vi "ALTS-2015 Convert Test Time format.vi"(8 "error in (no error)":errorcluster, 11 "String":string) -> (0 "error out":errorcluster, 3 "Test Time(YYYYMMDDHHMMSS)":string)   [LabVIEW 2013]
doc: "Copyright © 2005, Soliton Technologies.\nAll rights reserved."
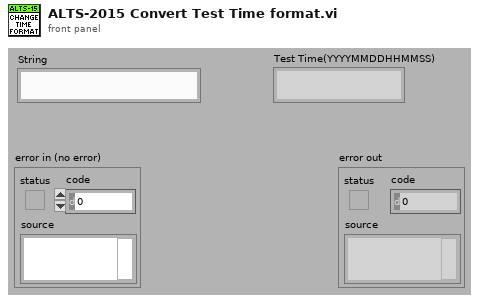
[diagram p1: front panel]
types:
  T1 = cluster{"YYYY":string, "MM":string, "DD":string, "HH":string, "Min MM":string, "SS":string}
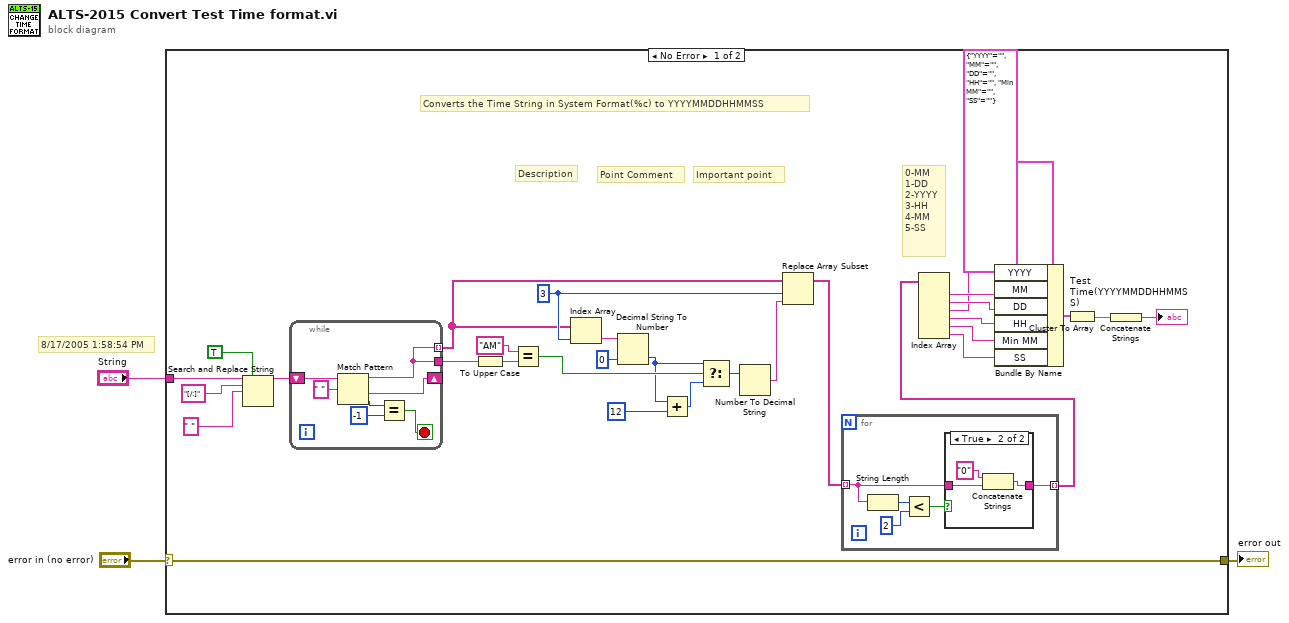
[diagram p0: block diagram]
diagram:
  # "8/17/2005 1:58:54 PM"
  n1 = case shown="No Error" "error in (no error)" {
    selector: "error in (no error)" -> [w34 w51]
    tunnel: [w34 w51] -> w2
    tunnel: "String" -> [w21 _]
    frame No Error {
      w31 = 3 ("index")
      # "Converts the Time String in System Format(%c) to YYYYMMDDHHMMSS"
      # "0-MM\n1-DD\n2-YYYY\n3-HH\n4-MM\n5-SS"
      # "Point Comment"
      # "Important point"
      # "Description"
      n2 = Search and Replace String(replace all?=TRUE ("replace all? (F)"), input string=w21, search string="[/:]", replace string=" " ("replace string (\"\")")) -> (result string=w20:string)  [unwired: 4 in, 3 out]
      n3 = while {
        shift-right: [w48] -> _
        shift-left: w20 -> [w50]
        tunnel: [w44] -> w17 mode=indexing
        tunnel: [w44] -> w5
        stop <- w45 stop-if-true
        n4 = Match Pattern(string=w50, regular expression=" ") -> (before substring=w44:string, after substring=w48:string, offset past match=w47:i32)  [unwired: 1 in, 1 out]
        n5 = Equal?(x=w47, y=-1) -> (x = y?=w45:bool)
      }
      n6 = To Upper Case(1:w5) -> (0:w33:string)
      n7 = Equal?(x="AM", y=w33) -> (x = y?=w28:bool)
      n8 = Index Array(array=w17, index=w31) -> (element=w30:string)
      n9 = Decimal String To Number(string=w30, default (0L)=0 ("default (0 I32)")) -> (number=w19:i32)  [unwired: 1 in, 1 out]
      n10 = Add(x=w19, y=12) -> (x+y=w27:i32)
      n11 = Select(t=w19, s=w28, f=w27) -> (s? t:f=w26:i32)
      n12 = Number To Decimal String(number=w26) -> (decimal integer string=w25:string)  [unwired: 1 in]
      n13 = Replace Array Subset(array=w17, new element=w25, index=w31) -> (w4:string[])
      n14 = for {
        tunnel: [w37] -> w16 mode=indexing
        tunnel: w4 -> [w36] mode=indexing
        n15 = String Length(string=w36) -> (length=w35:i32)
        n16 = Less?(x=w35, y=2) -> (x < y?=w38:bool)
        n17 = case shown="True" w38 {
          tunnel: w36 -> [w40 w42]
          tunnel: [w40 w41] -> w37
          frame False {
          }
          frame True {
            n18 = Concatenate Strings("0" ("string"), w42) -> (w41:string)
          }
        }
      }
      n19 = Index Array(array=w16) -> (element #1=w14:string, element #2=w13:string, element #3=w9:string, element #4=w12:string, element #5=w11:string, element #6=w10:string)  [unwired: 6 in]
      n20 = Bundle By Name(cluster=T1 {"YYYY"="", "MM"="", "DD"="", "HH"="", "Min MM"="", "SS"=""} ("input cluster"), "YYYY"=w9, "MM"=w14, "DD"=w13, "HH"=w12, "Min MM"=w11, "SS"=w10) -> (w8:T1)
      n21 = Cluster To Array(cluster=w8) -> (array=w7:string[])
      n22 = Concatenate Strings(w7) -> (→"Test Time(YYYYMMDDHHMMSS)":string)
    }
    frame Error {
    }
  }
  "error out" <- w2
